vi "SunplusDailyS2TMultiMachine.vi"() -> ()   [LabVIEW 2012]
uses:
  <vilib>/addons/database/Auxilliary.llb/DB Tools Cursor Type.ctl
  <vilib>/Utility/NIReport.llb/NI_report.lvclass
  <vilib>/addons/database/Connection.llb/DB Tools Open Connec (Path).vi
  <vilib>/addons/database/Connection.llb/Conn Execute.vi
  <vilib>/addons/database/Recordset.llb/Rec Fetch Recordset Data (R).vi
  <vilib>/addons/database/Recordset.llb/Rec Destroy - Connection.vi
  <vilib>/addons/database/_DB Variant To Data/Database Variant To Data.xnode
  <vilib>/addons/database/NI_Database_API.lvlib
  <vilib>/Utility/NIReport.llb/Excel/NI_Excel.lvclass
  <vilib>/Utility/SMTP/NI_SMTPEmail.lvlib
panel:
  out "error out":errorcluster
  in  "start (0, 0) 2":cluster{"start row":i32, "start column":i32}
  out "error out 2":errorcluster
  in  "MIME content-type (application/octet-stream)":string="application/octet-stream"
  out "error out 4":errorcluster
  in  "start (0, 0)":cluster{"start row":i32, "start column":i32}
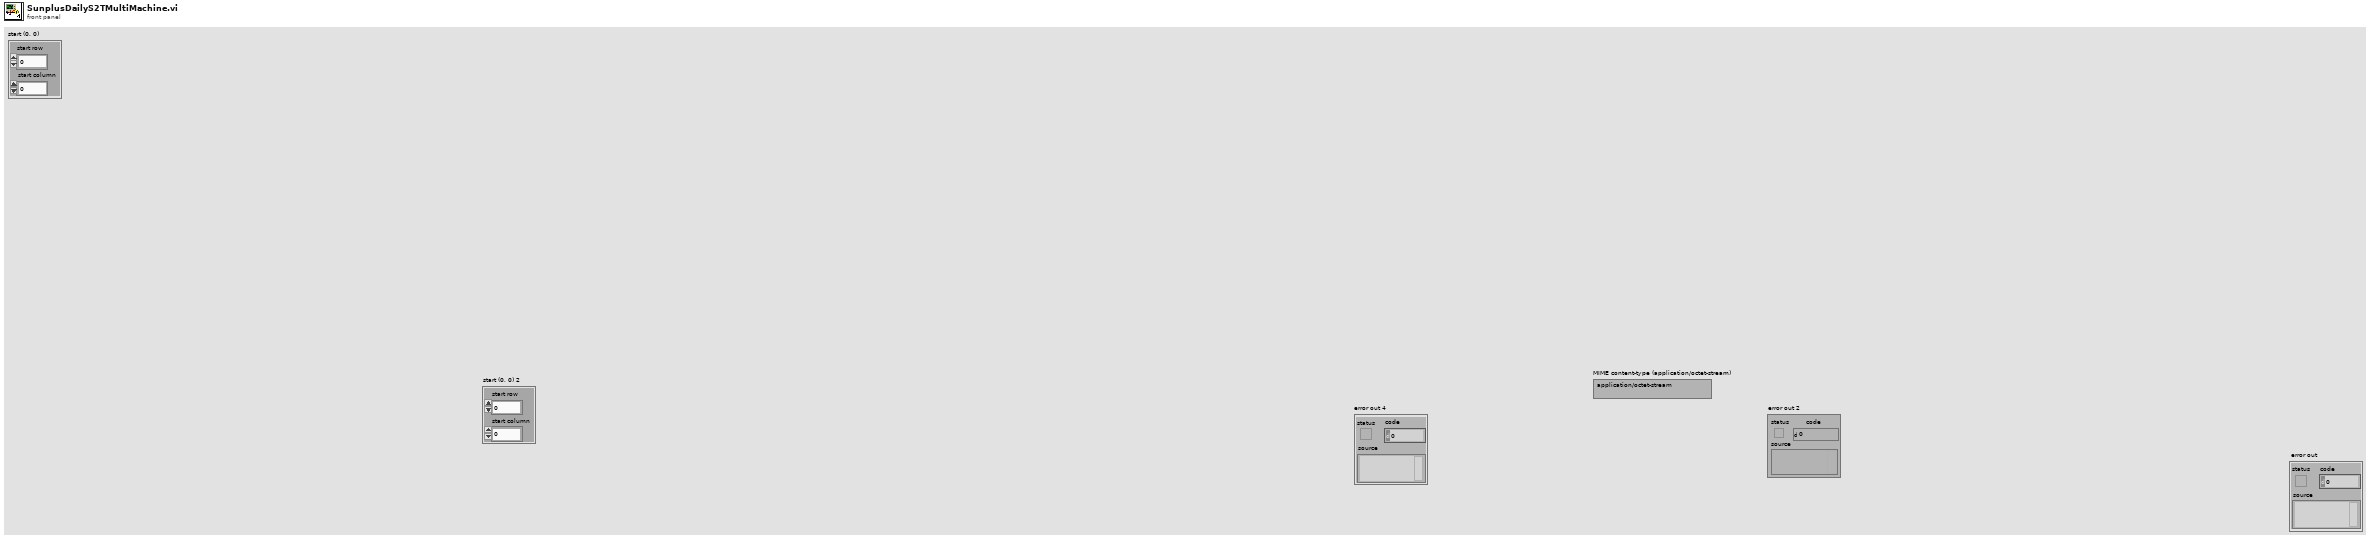
[diagram p1: front panel]
types:
  T1 = typedef "NI_Database_API.lvlib/DB Tools Cursor Type.ctl" = enum16{"forward-only", "keyset", "dynamic", "static"}
  T2 = enum16{"Standard Report", "HTML", "Word", "Excel"}
  T3 = typedef "NI_Database_API.lvlib/Conn ObjectReference.ctl" = refnum<k1>
  T4 = typedef "NI_Database_API.lvlib/Rec ObjectReference.ctl" = refnum<k1>
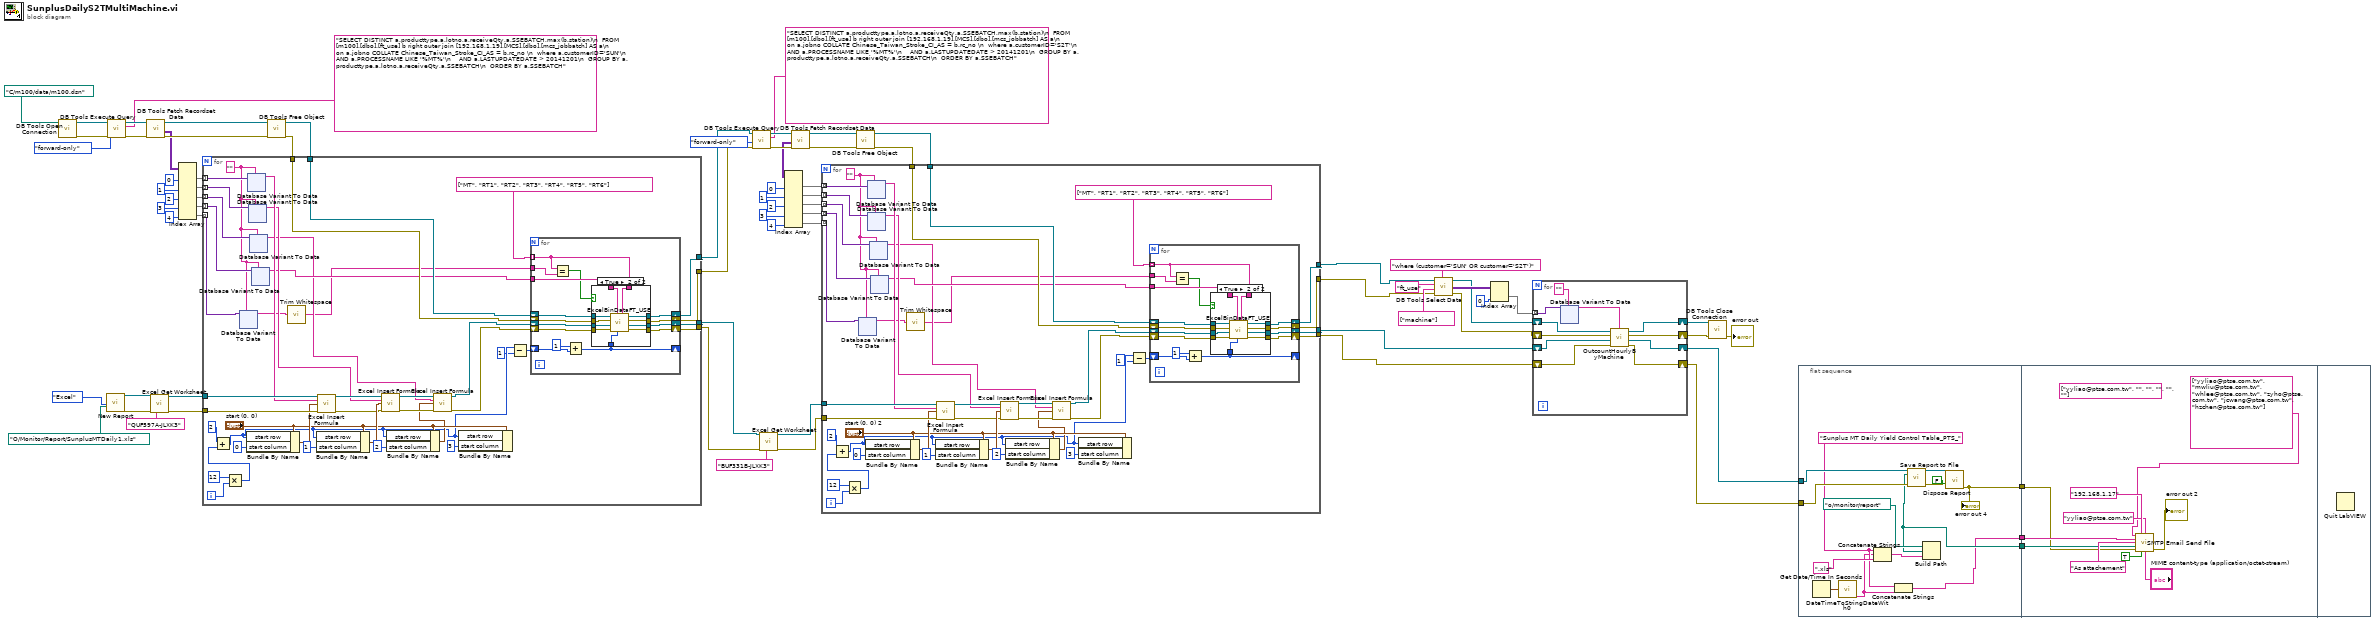
[diagram p0: block diagram]
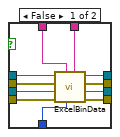
[diagram p2: hidden frame]
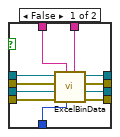
[diagram p3: hidden frame]
diagram:
  n1 = call-poly <vilib>:"DB Tools Open Connection.vi"("connection information"=path "C:/m100/data/m100.dsn") -> ("error out"=w67:errorcluster, "connection reference"=w68:T3)  [unwired: 7 in]
  n2 = call <vilib>:"New Report.vi"("report type"=T2."Excel" ("Report Type"), "template (empty)"=path "O:/Monitor/Report/SunplusMTDaily1.xls") -> ("report out"=w52:refnum<class "NI_report.lvclass">, "error out"=w51:errorcluster)  [unwired: 12 in]
  n3 = call-poly <vilib>:"DB Tools Execute Query.vi"("error in (no error)"=w67, "cursor type"=DB_Tools_Cursor_Type."forward-only", "SQL query"="SELECT DISTINCT a.producttype,a.lotno,a.receiveQty,a.SSEBATCH,max(b.station)\n  FROM [m100].[dbo].[ft_use] b right outer join [192.168.1.19].[MCS].[dbo].[mcs_jobbatch] AS a\n  on a.jobno COLLATE Chinese_Taiwan_Stroke_CI_AS = b.rc_no \n  where a.customerID='SUN'\n    AND a.PROCESSNAME LIKE '%MT%'\n    AND a.LASTUPDATEDATE > 20141201\n  GROUP BY a.producttype,a.lotno,a.receiveQty,a.SSEBATCH\n  ORDER BY a.SSEBATCH", "connection reference"=w68) -> ("error out"=w69:errorcluster, "recordset reference"=w70:T4)  [unwired: 4 in]
  n4 = call-poly <vilib>:"DB Tools Fetch Recordset Data.vi"("error in (no error)"=w69, "recordset reference"=w70) -> ("error out"=w71:errorcluster, "recordset data"=w64:variant[][], "recordset reference out"=w72:T4)  [unwired: 3 in]
  n5 = call <vilib>:"Excel Get Worksheet.vi"("report in"=w52, "error in (no error)"=w51, "name (\"\")"="QUF597A-JLXK3" ("name (\"\")")) -> ("report out"=w49:refnum<class "NI_report.lvclass">, "error out"=w48:errorcluster)  [unwired: 11 in]
  n6 = Index Array(array=w64, index (col) #1=0 ("disabled index (col)"), index (col) #2=1 ("index (col)"), index (col) #3=2 ("index (col)"), index (col) #4=3 ("index (col)"), index (col) #5=4 ("index (col)")) -> (element #1=w60:variant[], element #2=w59:variant[], element #3=w58:variant[], element #4=w54:variant[], element #5=w45:variant[])  [unwired: 5 in]
  n7 = call-poly <vilib>:"DB Tools Free Object.vi"("error in (no error)"=w71, "recordset reference"=w72) -> ("error out"=w57:errorcluster, "connection reference"=w56:T3)  [unwired: 8 in]
  n8 = for {
    tunnel: w60 -> [w117] mode=indexing
    tunnel: w59 -> [w116] mode=indexing
    tunnel: w58 -> [w115] mode=indexing
    tunnel: w57 -> [w92]
    tunnel: w56 -> [w93]
    tunnel: w54 -> [w114] mode=indexing
    tunnel: w49 -> [w113]
    tunnel: w48 -> [w112]
    tunnel: [w83] -> w21
    tunnel: [w82] -> w20
    tunnel: [w85] -> w39
    tunnel: [w84] -> w38
    tunnel: w45 -> [w79] mode=indexing
    i -> [w96]
    w78 = ""
    n9 = Multiply(x=12, y=w96) -> (x*y=w94:i32)
    n10 = Add(x=2, y=w94) -> (x+y=w89:i32)
    n11 = xnode "Database Variant To Data"("database variant"=w79, "type"=w78) -> ("data"=w77:string)  [unwired: 1 in, 1 out]
    n12 = Bundle By Name(cluster="start (0, 0)", "start row"=w89, "start column"=0) -> (w111:cluster{"start row":i32, "start column":i32})
    n13 = xnode "Database Variant To Data"("database variant"=w117, "type"=w78) -> ("data"=w108:string)  [unwired: 1 in, 1 out]
    n14 = xnode "Database Variant To Data"("database variant"=w116, "type"=w78) -> ("data"=w103:string)  [unwired: 1 in, 1 out]
    n15 = xnode "Database Variant To Data"("database variant"=w115, "type"=w78) -> ("data"=w80:string)  [unwired: 1 in, 1 out]
    n16 = xnode "Database Variant To Data"("database variant"=w114, "type"=w78) -> ("data"=w86:string)  [unwired: 1 in, 1 out]
    n17 = call <vilib>:"Trim Whitespace.vi"("string"=w77) -> ("trimmed string"=w76:string)  [unwired: 1 in]
    n18 = Bundle By Name(cluster="start (0, 0)", "start row"=w89, "start column"=1) -> (w106:cluster{"start row":i32, "start column":i32})
    n19 = call <vilib>:"Excel Insert Formula.vi"("report in"=w113, "formula"=w108, "start (0, 0)"=w111, "error in (no error)"=w112) -> ("report out"=w105:refnum<class "NI_report.lvclass">, "error out"=w104:errorcluster)  [unwired: 10 in]
    n20 = call <vilib>:"Excel Insert Formula.vi"("report in"=w105, "formula"=w103, "start (0, 0)"=w106, "error in (no error)"=w104) -> ("report out"=w101:refnum<class "NI_report.lvclass">, "error out"=w100:errorcluster)  [unwired: 10 in]
    n21 = Bundle By Name(cluster="start (0, 0)", "start row"=w89, "start column"=2) -> (w97:cluster{"start row":i32, "start column":i32})
    n22 = call <vilib>:"Excel Insert Formula.vi"("report in"=w101, "formula"=w80, "start (0, 0)"=w97, "error in (no error)"=w100) -> ("report out"=w91:refnum<class "NI_report.lvclass">, "error out"=w90:errorcluster)  [unwired: 10 in]
    n23 = Bundle By Name(cluster="start (0, 0)", "start row"=w89, "start column"=3) -> ()  [unwired: 1 out]
    n24 = Subtract(x=w89, y=1) -> (x-y=w87:i32)
    n25 = for {
      shift-right: [w163] -> w85
      shift-left: w93 -> [w156]
      shift-right: [w162] -> w84
      shift-left: w92 -> [w155]
      shift-right: [w161] -> w83
      shift-left: w91 -> [w154]
      shift-right: [w160] -> w82
      shift-left: w90 -> [w153]
      shift-right: [w159] -> _
      shift-left: w87 -> [w158]
      tunnel: w86 -> [w157]
      tunnel: string[] ["MT", "RT1", "RT2", "RT3", "RT4", "RT5", "RT6"] ("Array") -> [w151] mode=indexing
      tunnel: w76 -> [w152]
      n26 = Equal?(x=w151, y=w152) -> (x = y?=w150:bool)
      n27 = Add(x=1, y=w158) -> (x+y=w159:i32)
      n28 = case shown="True" w150 {
        tunnel: [w175 w181] -> w163
        tunnel: [w174 w180] -> w162
        tunnel: [w173 w179] -> w161
        tunnel: [w172 w178] -> w160
        tunnel: w159 -> [w171 w186]
        tunnel: w157 -> [w170 w177]
        tunnel: w156 -> [w169 w185]
        tunnel: w155 -> [w168 w184]
        tunnel: w154 -> [w167 w183]
        tunnel: w153 -> [w166 w182]
        tunnel: w151 -> [w165 w176]
        frame False {
          n29 = call "ExcelBinData.vi"("step"=w165, "start row"=w171, "jobno"=w170, "error in (no error) 2"=w166, "report in"=w167, "error in (no error)"=w168, "connection reference 2"=w169) -> ("error out 2"=w172:errorcluster, "report out"=w173:refnum<class "NI_report.lvclass">, "error out"=w174:errorcluster, "connection reference"=w175:T3)  [unwired: 1 in]
        }
        frame True {
          n30 = call "ExcelBinDataFT_USE.vi"("step"=w176, "start row"=w186, "jobno"=w177, "error in (no error) 2"=w182, "report in"=w183, "error in (no error)"=w184, "connection reference 2"=w185) -> ("error out 2"=w178:errorcluster, "report out"=w179:refnum<class "NI_report.lvclass">, "error out"=w180:errorcluster, "connection reference"=w181:T3)  [unwired: 1 in]
        }
      }
    }
  }
  n31 = call-poly <vilib>:"DB Tools Execute Query.vi"("error in (no error)"=w38, "cursor type"=DB_Tools_Cursor_Type."forward-only", "SQL query"="SELECT DISTINCT a.producttype,a.lotno,a.receiveQty,a.SSEBATCH,max(b.station)\n  FROM [m100].[dbo].[ft_use] b right outer join [192.168.1.19].[MCS].[dbo].[mcs_jobbatch] AS a\n  on a.jobno COLLATE Chinese_Taiwan_Stroke_CI_AS = b.rc_no \n  where a.customerID='S2T'\n    AND a.PROCESSNAME LIKE '%MT%'\n    AND a.LASTUPDATEDATE > 20141201\n  GROUP BY a.producttype,a.lotno,a.receiveQty,a.SSEBATCH\n  ORDER BY a.SSEBATCH", "connection reference"=w39) -> ("error out"=w41:errorcluster, "recordset reference"=w42:T4)  [unwired: 4 in]
  n32 = call <vilib>:"Excel Get Worksheet.vi"("report in"=w21, "error in (no error)"=w20, "name (\"\")"="BUF331B-JLXK3" ("name (\"\")")) -> ("report out"=w23:refnum<class "NI_report.lvclass">, "error out"=w22:errorcluster)  [unwired: 11 in]
  n33 = call-poly <vilib>:"DB Tools Fetch Recordset Data.vi"("error in (no error)"=w41, "recordset reference"=w42) -> ("error out"=w43:errorcluster, "recordset data"=w32:variant[][], "recordset reference out"=w44:T4)  [unwired: 3 in]
  n34 = Index Array(array=w32, index (col) #1=0 ("disabled index (col)"), index (col) #2=1 ("index (col)"), index (col) #3=2 ("index (col)"), index (col) #4=3 ("index (col)"), index (col) #5=4 ("index (col)")) -> (element #1=w30:variant[], element #2=w29:variant[], element #3=w28:variant[], element #4=w27:variant[], element #5=w26:variant[])  [unwired: 5 in]
  n35 = call-poly <vilib>:"DB Tools Free Object.vi"("error in (no error)"=w43, "recordset reference"=w44) -> ("error out"=w25:errorcluster, "connection reference"=w24:T3)  [unwired: 8 in]
  n36 = for {
    tunnel: w30 -> [w356] mode=indexing
    tunnel: w29 -> [w355] mode=indexing
    tunnel: w28 -> [w354] mode=indexing
    tunnel: w25 -> [w331]
    tunnel: w24 -> [w332]
    tunnel: w27 -> [w353] mode=indexing
    tunnel: w23 -> [w352]
    tunnel: w22 -> [w351]
    tunnel: [w322] -> w9
    tunnel: [w321] -> w8
    tunnel: [w324] -> w10
    tunnel: [w323] -> w11
    tunnel: w26 -> [w318] mode=indexing
    i -> [w335]
    w317 = ""
    n37 = Multiply(x=12, y=w335) -> (x*y=w333:i32)
    n38 = Add(x=2, y=w333) -> (x+y=w328:i32)
    n39 = xnode "Database Variant To Data"("database variant"=w318, "type"=w317) -> ("data"=w316:string)  [unwired: 1 in, 1 out]
    n40 = Bundle By Name(cluster="start (0, 0) 2", "start row"=w328, "start column"=0) -> (w350:cluster{"start row":i32, "start column":i32})
    n41 = xnode "Database Variant To Data"("database variant"=w356, "type"=w317) -> ("data"=w347:string)  [unwired: 1 in, 1 out]
    n42 = xnode "Database Variant To Data"("database variant"=w355, "type"=w317) -> ("data"=w342:string)  [unwired: 1 in, 1 out]
    n43 = xnode "Database Variant To Data"("database variant"=w354, "type"=w317) -> ("data"=w319:string)  [unwired: 1 in, 1 out]
    n44 = xnode "Database Variant To Data"("database variant"=w353, "type"=w317) -> ("data"=w325:string)  [unwired: 1 in, 1 out]
    n45 = call <vilib>:"Trim Whitespace.vi"("string"=w316) -> ("trimmed string"=w315:string)  [unwired: 1 in]
    n46 = Bundle By Name(cluster="start (0, 0) 2", "start row"=w328, "start column"=1) -> (w345:cluster{"start row":i32, "start column":i32})
    n47 = call <vilib>:"Excel Insert Formula.vi"("report in"=w352, "formula"=w347, "start (0, 0)"=w350, "error in (no error)"=w351) -> ("report out"=w344:refnum<class "NI_report.lvclass">, "error out"=w343:errorcluster)  [unwired: 10 in]
    n48 = call <vilib>:"Excel Insert Formula.vi"("report in"=w344, "formula"=w342, "start (0, 0)"=w345, "error in (no error)"=w343) -> ("report out"=w340:refnum<class "NI_report.lvclass">, "error out"=w339:errorcluster)  [unwired: 10 in]
    n49 = Bundle By Name(cluster="start (0, 0) 2", "start row"=w328, "start column"=2) -> (w336:cluster{"start row":i32, "start column":i32})
    n50 = call <vilib>:"Excel Insert Formula.vi"("report in"=w340, "formula"=w319, "start (0, 0)"=w336, "error in (no error)"=w339) -> ("report out"=w330:refnum<class "NI_report.lvclass">, "error out"=w329:errorcluster)  [unwired: 10 in]
    n51 = Bundle By Name(cluster="start (0, 0) 2", "start row"=w328, "start column"=3) -> ()  [unwired: 1 out]
    n52 = Subtract(x=w328, y=1) -> (x-y=w326:i32)
    n53 = for {
      shift-right: [w402] -> w324
      shift-left: w332 -> [w395]
      shift-right: [w401] -> w323
      shift-left: w331 -> [w394]
      shift-right: [w400] -> w322
      shift-left: w330 -> [w393]
      shift-right: [w399] -> w321
      shift-left: w329 -> [w392]
      shift-right: [w398] -> _
      shift-left: w326 -> [w397]
      tunnel: w325 -> [w396]
      tunnel: string[] ["MT", "RT1", "RT2", "RT3", "RT4", "RT5", "RT6"] ("Array") -> [w390] mode=indexing
      tunnel: w315 -> [w391]
      n54 = Equal?(x=w390, y=w391) -> (x = y?=w389:bool)
      n55 = Add(x=1, y=w397) -> (x+y=w398:i32)
      n56 = case shown="True" w389 {
        tunnel: [w414 w420] -> w402
        tunnel: [w413 w419] -> w401
        tunnel: [w412 w418] -> w400
        tunnel: [w411 w417] -> w399
        tunnel: w398 -> [w410 w425]
        tunnel: w396 -> [w409 w416]
        tunnel: w395 -> [w408 w424]
        tunnel: w394 -> [w407 w423]
        tunnel: w393 -> [w406 w422]
        tunnel: w392 -> [w405 w421]
        tunnel: w390 -> [w404 w415]
        frame False {
          n57 = call "ExcelBinData.vi"("step"=w404, "start row"=w410, "jobno"=w409, "error in (no error) 2"=w405, "report in"=w406, "error in (no error)"=w407, "connection reference 2"=w408) -> ("error out 2"=w411:errorcluster, "report out"=w412:refnum<class "NI_report.lvclass">, "error out"=w413:errorcluster, "connection reference"=w414:T3)  [unwired: 1 in]
        }
        frame True {
          n58 = call "ExcelBinDataFT_USE.vi"("step"=w415, "start row"=w425, "jobno"=w416, "error in (no error) 2"=w421, "report in"=w422, "error in (no error)"=w423, "connection reference 2"=w424) -> ("error out 2"=w417:errorcluster, "report out"=w418:refnum<class "NI_report.lvclass">, "error out"=w419:errorcluster, "connection reference"=w420:T3)  [unwired: 1 in]
        }
      }
    }
  }
  n59 = call <vilib>:"DB Tools Select Data.vi"("condition"="where (customer='SUN' OR customer='S2T')", "error in (no error)"=w11, "columns"=string[] ["machine"], "table"="ft_use", "connection reference"=w10) -> ("error out"=w12:errorcluster, "data"=w16:variant[][], "connection reference out"=w13:T3)  [unwired: 1 in]
  n60 = Index Array(array=w16, index (col)=0 ("disabled index (col)")) -> (element=w15:variant[])  [unwired: 1 in]
  n61 = for {
    tunnel: w15 -> [w563] mode=indexing
    shift-right: [w557] -> w6
    shift-left: w13 -> [w555]
    shift-right: [w556] -> w5
    shift-left: w12 -> [w554]
    shift-right: [w560] -> w4
    shift-left: w9 -> [w564]
    shift-right: [w559] -> w3
    shift-left: w8 -> [w558]
    n62 = xnode "Database Variant To Data"("database variant"=w563, "type"="") -> ("data"=w561:string)  [unwired: 1 in, 1 out]
    n63 = call "OutcountHourlyByMachine.vi"("Machine"=w561, "error in (no error) 2"=w558, "report in"=w564, "error in (no error)"=w554, "connection reference"=w555) -> ("error in (no error) 3"=w559:errorcluster, "report in 2"=w560:refnum<class "NI_report.lvclass">, "error out"=w556:errorcluster, "connection reference 2"=w557:T3)  [unwired: 3 in]
  }
  n64 = call <vilib>:"DB Tools Close Connection.vi"("error in (no error)"=w5, "connection reference"=w6) -> ("error out"=→"error out":errorcluster)  [unwired: 5 in]
  n65 = flat-sequence {
    tunnel: w4 -> [w606]
    tunnel: w3 -> [w605]
    tunnel: [w597] -> w75
    tunnel: [w601] -> w74
    tunnel: [w600] -> w73
    tunnel: w75 -> [w614]
    tunnel: w74 -> [w613]
    tunnel: w73 -> [w612]
    frame #0 {
      w599 = "Sunplus MT Daily Yield Control Table_PTS_" ("string")
      n66 = Get Date/Time In Seconds() -> (seconds since 1Jan1904=w603:timestamp)
      n67 = call "DateTimeToStringDateWith0.vi"("time stamp"=w603) -> ("Dateyyyymmdd"=w598:string)  [unwired: 9 in, 1 out]
      n68 = Concatenate Strings(w599, w598, ".xls" ("string")) -> (w602:string)
      n69 = Concatenate Strings(w599, w598) -> (w597:string)
      n70 = Build Path(base path=path "o:/monitor/report", name or relative path=w602) -> (appended path=w601:path)
      n71 = call-dynamic "Save Report to File.vi"("report in"=w606, "report file path"=w601, "error in (no error)"=w605) -> ("report out"=w608:refnum<class "NI_report.lvclass">, "error out"=w607:errorcluster)  [unwired: 11 in]
      n72 = call-dynamic "Dispose Report.vi"("report in"=w608, "save changes? (F)"=FALSE, "error in (no error)"=w607) -> ("error out"=w600:errorcluster)  [unwired: 12 in]
      "error out 4" <- w600
    }
    frame #1 {
      (unwired) string[] ["yyliao@ptse.com.tw", "", "", "", "", ""] ("recipients")
      n73 = call <vilib>:"SMTP Email Send File.vi"("recipients"=string[] ["yyliao@ptse.com.tw", "mwliu@ptse.com.tw", "whlee@ptse.com.tw", "zyho@ptse.com.tw", "jcwang@ptse.com.tw", "hzchen@ptse.com.tw"], "mail server"="192.168.1.17", "return address"="yyliao@ptse.com.tw", "subject ([No Subject])"=w614, "message"="As attachement", "file path"=w613, "error in (no error)"=w612, "binary? (F)"=TRUE, "MIME content-type (application/octet-stream)"="MIME content-type (application/octet-stream)") -> ("error out"=→"error out 2":errorcluster)  [unwired: 5 in, 1 out]
    }
    frame #2 {
      n74 = Quit LabVIEW() -> ()  [unwired: 1 in]
    }
  }
